vi "02_ui_plot_window.vi"() -> ()   [LabVIEW 2025]
uses:
  4c7a61b9-d50a-4fa5-8b88-644507a3af04.vi
  74ea501e-f43b-483f-8511-84a735437533.vi
  166e0385-1291-4ee6-a608-8b02bdaae3d2.vi
  b1158e5f-e22e-42fa-9d41-9ea4e4d0b9e3.vi
  31b119fa-27fe-4ebe-809c-2da1a8fd4d96.vi
  13143f16-a64c-4a8d-9511-2945b8db9dc5.vi
  9c1d92a2-1c85-4809-97a6-d36bf52cbad7.vi
  d684625a-03c4-4daf-8e9e-674a236ebb3e.vi
  fb960f78-e1fe-4b5d-8417-6d8be925c5cf.vi
  c135c75a-78bf-4448-8d92-d4bbbd51cd11.vi
  <vilib>/Utility/config.llb/Read Key (U32).vi
  <vilib>/Utility/config.llb/Read Key (Boolean).vi
  <vilib>/Utility/config.llb/Read Key (String).vi
  <vilib>/Utility/config.llb/Write Key (U32).vi
  <vilib>/Utility/config.llb/Write Key (Boolean).vi
  <vilib>/Utility/config.llb/Write Key (String).vi
  00_global_variables.vi
  <vilib>/Utility/config.llb/NI_LVConfig.lvlib
panel:
  out "loaded_config_path":path
  out "loaded_config_filename":string caption="Recent File"
  in  "open_config_plot_0":bool
  in  "safe_config_as_plot_0":bool
  in  "safe_config_plot_0":bool
  in  "select_plot_5":string(combo)="2"
  in  "select_plot_4":string(combo)="2"
  out "cursor_p5_1_prefix":string
  out "cursor_p4_1_prefix":string
  out "cursor_p5_2_prefix":string
  out "cursor_p4_2_prefix":string
  out "cursor_p5_2":dbl format="%#_6f"
  in  "color_picker_5":u32(colorbox)=14811391
  out "cursor_p5_1":dbl format="%#_6f"
  in  "enable_plot_5":bool caption="S11 - Imaginary"
  out "cursor_p4_2":dbl format="%#_6f"
  in  "color_picker_4":u32(colorbox)=49352
  out "cursor_p4_1":dbl format="%#_6f"
  in  "enable_plot_4":bool caption="S11 - Imaginary"
  in  "select_plot_3":string(combo)="2"
  in  "select_plot_2":string(combo)="2"
  in  "select_plot_1":string(combo)="2"
  in  "select_plot_0":string(combo)="2"
  out "cursor_p3_1_prefix":string
  out "cursor_p2_1_prefix":string
  out "cursor_p1_1_prefix":string
  out "cursor_p0_1_prefix":string
  out "cursor_p3_2_prefix":string
  out "cursor_p2_2_prefix":string
  out "cursor_p1_2_prefix":string
  out "cursor_p0_2_prefix":string
  out "cursor_p3_2":dbl format="%#_6f"
  in  "color_picker_3":u32(colorbox)=14468608
  out "cursor_p3_1":dbl format="%#_6f"
  in  "enable_plot_3":bool caption="S11 - Imaginary"
  out "cursor_p2_2":dbl format="%#_6f"
  in  "color_picker_2":u32(colorbox)=39219
  out "cursor_p2_1":dbl format="%#_6f"
  in  "enable_plot_2":bool caption="S11 - Imaginary"
  out "cursor_p1_2":dbl format="%#_6f"
  out "cursor_p0_2":dbl format="%#_6f"
  out "cursor_p0_freq_2":string caption="Frequenz"
  out "cursor_p0_wavel_2":dbl caption="Frequenz"
  out "cursor_p0_wavel_1":dbl caption="Frequenz"
  in  "color_picker_1":u32(colorbox)=14423100
  in  "color_picker_0":u32(colorbox)=26316
  out "cursor_p0_freq_1":string caption="Frequenz"
  out "cursor_p1_1":dbl format="%#_6f"
  out "cursor_p0_1":dbl format="%#_6f"
  in  "enable_plot_1":bool caption="S11 - Imaginary"
  in  "enable_plot_0":bool=TRUE
  out "plot_0":cluster{"array type (2D Dbl)":dbl[], dbl[]}[](graph)
  # "Cursor 2"
  # "Cursor 1"
  # "Hz"
  # "Frequency"
  # "Hz"
  # "Wavelength"
  # "m"
  # "m"
  # "Configuration"
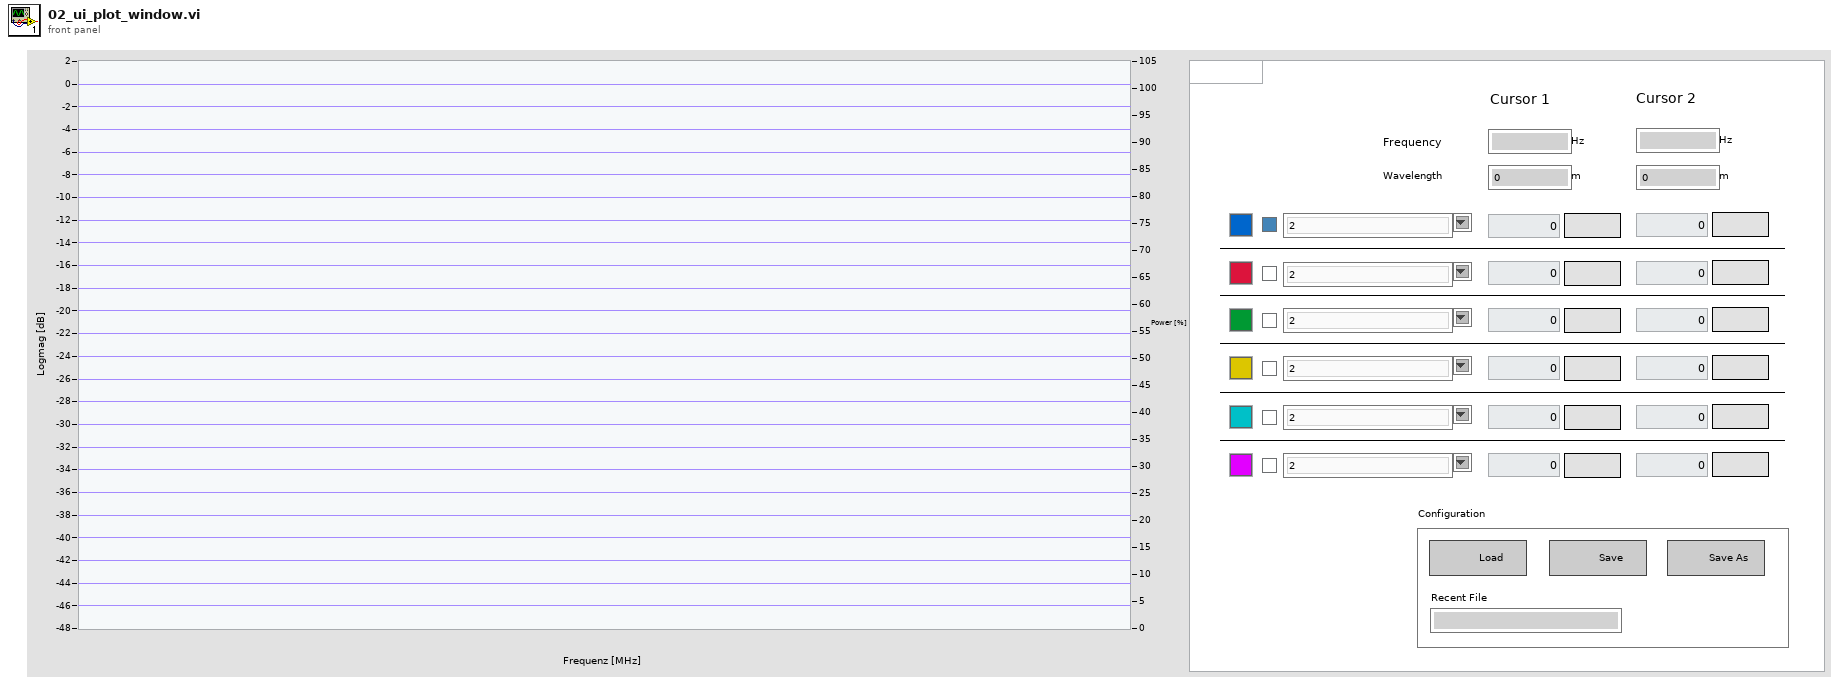
[diagram p1: front panel]
types:
  T1 = typedef "NI_LVConfig.lvlib/Config Data RefNum.ctl" = refnum<k1>
  T2 = typedef "LVComboBoxStrsAndValuesArrayTypeDef.ctl" = cluster{"String":string, "Value":string}[]
  T3 = cluster{"freq_array":dbl[], "data_array":dbl[]}[]
  T4 = cluster{"y_scale_id":u32, "unit":string, "prefix_enable":bool, "plot_id":u32}[]
  T5 = cluster{"y_scale_id":u32, "unit":string, "prefix_enable":bool, "plot_id":u32}
  T6 = typedef "LVCursorListTypeDef.ctl" = cluster{"Name":string, "Color":u32, "Style":u8, "Point Style":u8, "Name Visible":bool, "Allow Drag":bool, "Cursor Mode":u32, "Plot":i32, "Index":i32, "Position":cluster{"X":dbl, "Y":dbl}, "X Scale":u32, "Y Scale":u32, "Watch Plots":i32[], "Watch All Plots":bool, "Plot Area":i32, "Label Offset":cluster{"X":dbl, "Y":dbl}}[]
  T7 = cluster{"cursor_data":dbl[], "frequency":string, "wavelength_m":dbl}
  T8 = cluster{"cursor_0_color":u32, "cursor_1_color":u32}
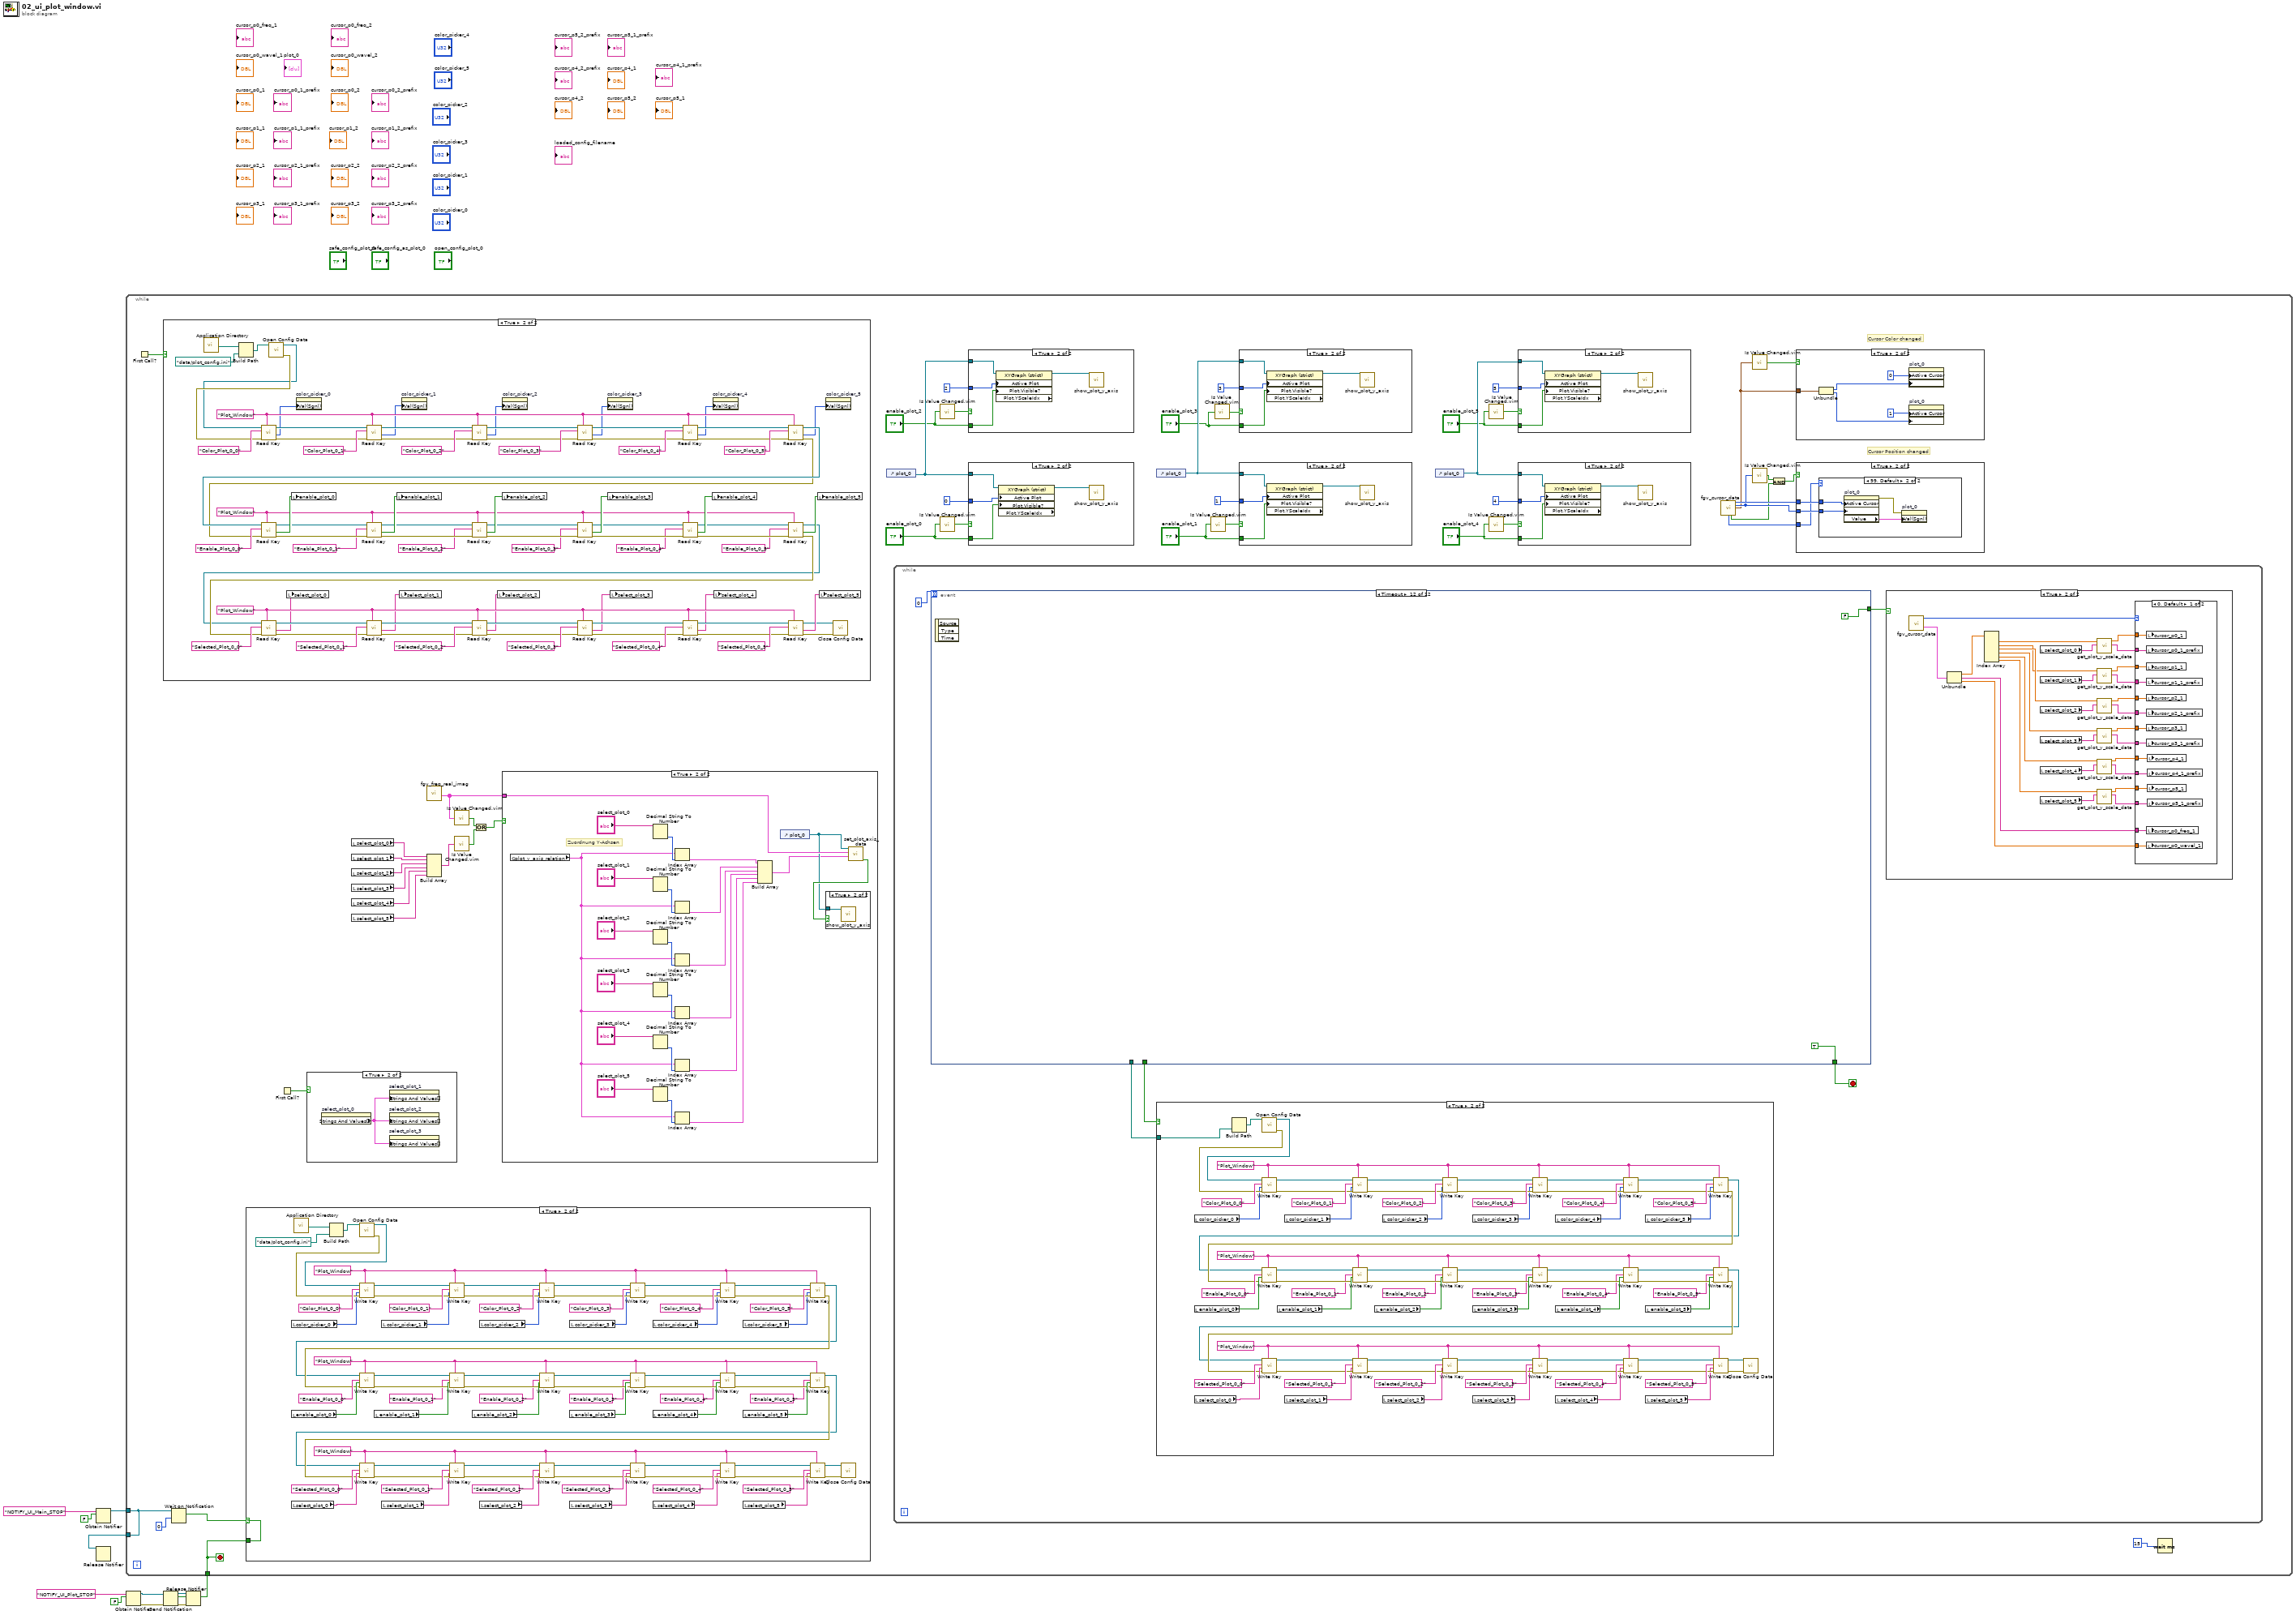
[diagram p0: block diagram]
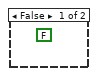
[diagram p11: hidden frame]
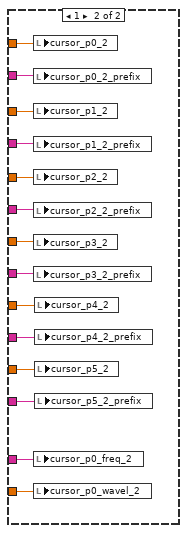
[diagram p18: hidden frame]
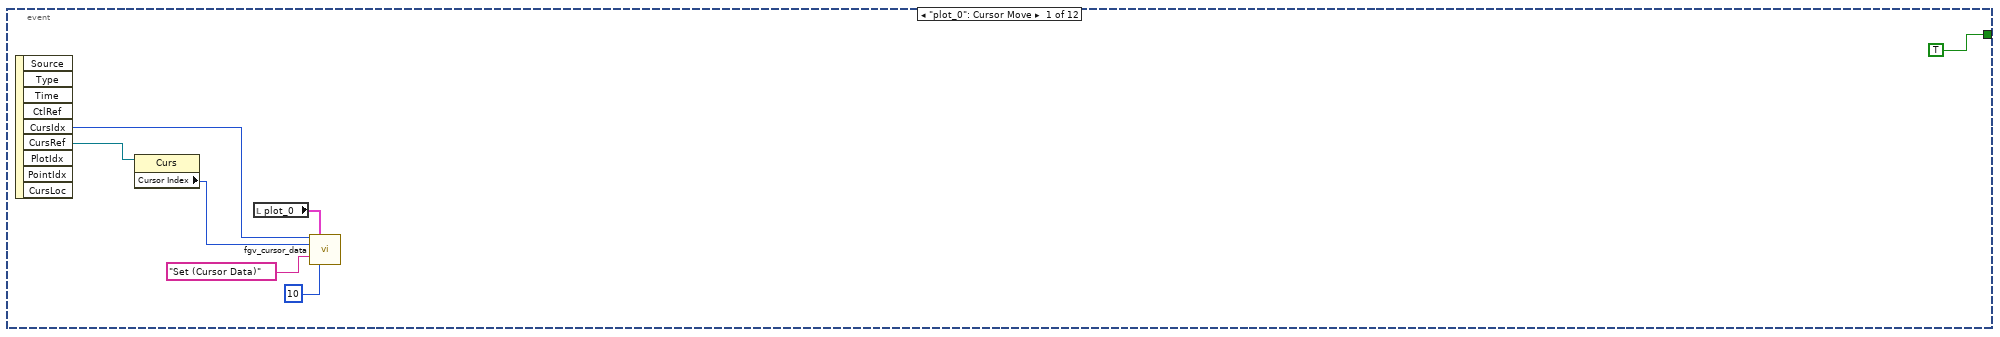
[diagram p19: hidden frame]
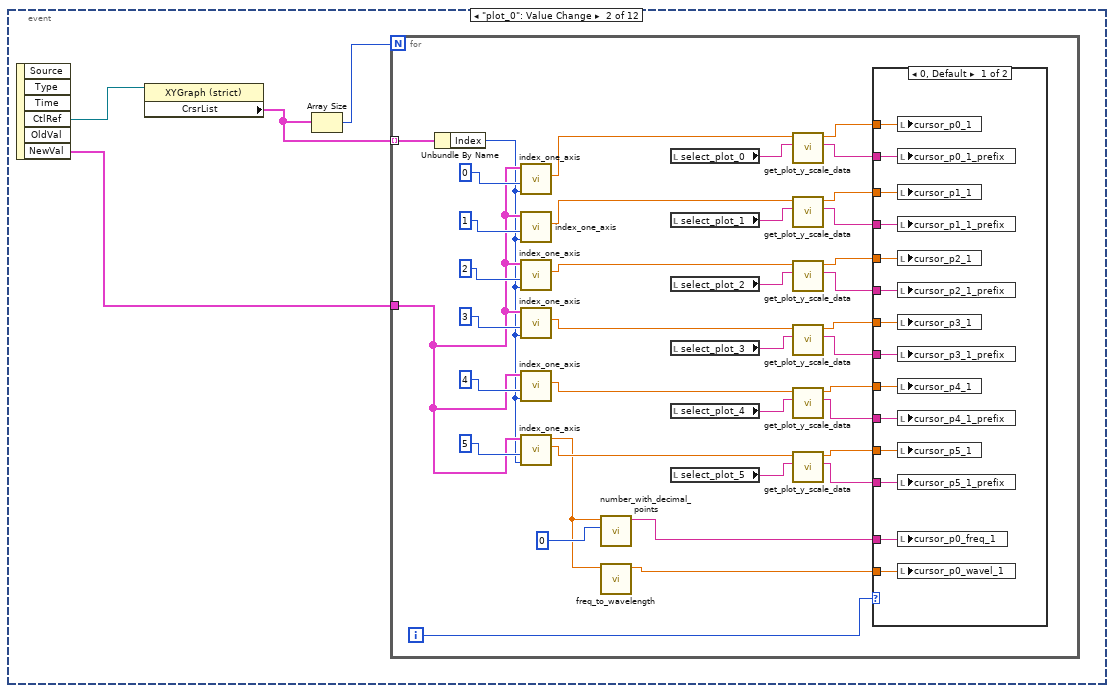
[diagram p20: hidden frame]
diagram:
  n1 = Obtain Notifier(name (unnamed)="NOTIFY_UI_Main_STOP", notification data type=FALSE) -> (notifier out=w9:refnum<notifier>)  [unwired: 2 in, 2 out]
  n2 = while {
    tunnel: w9 -> [w35]
    tunnel: [w35] -> w8
    tunnel: [w21] -> w1
    stop <- w21 stop-if-true
    # "Cursor Color changed"
    # "Cursor Position changed"
    n3 = First Call?() -> (First Call?: T/F=w20:bool)
    n4 = case shown="True" w20 {
      frame False {
      }
      frame True {
        w173 = "Plot_Window" ("section")
        w208 = "Plot_Window" ("section")
        w215 = "Plot_Window" ("section")
        n5 = call <vilib>:"Application Directory.vi"() -> ("Application Directory"=w158:path)
        n6 = Build Path(base path=w158, name or relative path=path "data/plot_config.ini") -> (appended path=w164:path)
        n7 = call <vilib>:"Open Config Data.vi"("configuration file path"=w164) -> ("error out"=w162:errorcluster, "refnum"=w161:T1)  [unwired: 8 in, 1 out]
        n8 = call-poly <vilib>:"Read Key.vi"("section"=w215, "error in (no error)"=w162, "key"="Color_Plot_0_0", "refnum"=w161) -> ("error out"=w228:errorcluster, "value"=w157:u32, "refnum out"=w229:T1)  [unwired: 4 in, 1 out]
        n9 = property on="color_picker_0" class="ColBox"("Val(Sgnl)"=w157) -> ()  [unwired: 2 in, 2 out]
        n10 = call-poly <vilib>:"Read Key.vi"("section"=w215, "error in (no error)"=w228, "key"="Color_Plot_0_1", "refnum"=w229) -> ("error out"=w225:errorcluster, "value"=w156:u32, "refnum out"=w226:T1)  [unwired: 4 in, 1 out]
        n11 = property on="color_picker_1" class="ColBox"("Val(Sgnl)"=w156) -> ()  [unwired: 2 in, 2 out]
        n12 = call-poly <vilib>:"Read Key.vi"("section"=w215, "error in (no error)"=w225, "key"="Color_Plot_0_2", "refnum"=w226) -> ("error out"=w222:errorcluster, "value"=w152:u32, "refnum out"=w223:T1)  [unwired: 4 in, 1 out]
        n13 = property on="color_picker_2" class="ColBox"("Val(Sgnl)"=w152) -> ()  [unwired: 2 in, 2 out]
        n14 = call-poly <vilib>:"Read Key.vi"("section"=w215, "error in (no error)"=w222, "key"="Color_Plot_0_3", "refnum"=w223) -> ("error out"=w219:errorcluster, "value"=w153:u32, "refnum out"=w220:T1)  [unwired: 4 in, 1 out]
        n15 = property on="color_picker_3" class="ColBox"("Val(Sgnl)"=w153) -> ()  [unwired: 2 in, 2 out]
        n16 = call-poly <vilib>:"Read Key.vi"("section"=w215, "error in (no error)"=w219, "key"="Color_Plot_0_4", "refnum"=w220) -> ("error out"=w217:errorcluster, "value"=w154:u32, "refnum out"=w216:T1)  [unwired: 4 in, 1 out]
        n17 = property on="color_picker_4" class="ColBox"("Val(Sgnl)"=w154) -> ()  [unwired: 2 in, 2 out]
        n18 = call-poly <vilib>:"Read Key.vi"("section"=w215, "error in (no error)"=w217, "key"="Color_Plot_0_5", "refnum"=w216) -> ("error out"=w190:errorcluster, "value"=w155:u32, "refnum out"=w191:T1)  [unwired: 4 in, 1 out]
        n19 = call-poly <vilib>:"Read Key.vi"("section"=w208, "error in (no error)"=w190, "key"="Enable_Plot_0_0", "refnum"=w191) -> ("error out"=w195:errorcluster, "value"=w209:bool, "refnum out"=w194:T1)  [unwired: 4 in, 1 out]
        n20 = local write "enable_plot_0"(w209) -> ()
        n21 = call-poly <vilib>:"Read Key.vi"("section"=w208, "error in (no error)"=w195, "key"="Enable_Plot_0_1", "refnum"=w194) -> ("error out"=w198:errorcluster, "value"=w210:bool, "refnum out"=w197:T1)  [unwired: 4 in, 1 out]
        n22 = local write "enable_plot_1"(w210) -> ()
        n23 = call-poly <vilib>:"Read Key.vi"("section"=w208, "error in (no error)"=w198, "key"="Enable_Plot_0_2", "refnum"=w197) -> ("error out"=w201:errorcluster, "value"=w211:bool, "refnum out"=w200:T1)  [unwired: 4 in, 1 out]
        n24 = local write "enable_plot_2"(w211) -> ()
        n25 = call-poly <vilib>:"Read Key.vi"("section"=w208, "error in (no error)"=w201, "key"="Enable_Plot_0_3", "refnum"=w200) -> ("error out"=w204:errorcluster, "value"=w212:bool, "refnum out"=w203:T1)  [unwired: 4 in, 1 out]
        n26 = local write "enable_plot_3"(w212) -> ()
        n27 = call-poly <vilib>:"Read Key.vi"("section"=w208, "error in (no error)"=w204, "key"="Enable_Plot_0_4", "refnum"=w203) -> ("error out"=w206:errorcluster, "value"=w213:bool, "refnum out"=w207:T1)  [unwired: 4 in, 1 out]
        n28 = local write "enable_plot_4"(w213) -> ()
        n29 = call-poly <vilib>:"Read Key.vi"("section"=w208, "error in (no error)"=w206, "key"="Enable_Plot_0_5", "refnum"=w207) -> ("error out"=w166:errorcluster, "value"=w214:bool, "refnum out"=w165:T1)  [unwired: 4 in, 1 out]
        n30 = call-poly <vilib>:"Read Key.vi"("section"=w173, "error in (no error)"=w166, "key"="Selected_Plot_0_0", "refnum"=w165) -> ("error out"=w186:errorcluster, "value"=w172:string, "refnum out"=w187:T1)  [unwired: 4 in, 1 out]
        n31 = local write "select_plot_0"(w172) -> ()
        n32 = call-poly <vilib>:"Read Key.vi"("section"=w173, "error in (no error)"=w186, "key"="Selected_Plot_0_1", "refnum"=w187) -> ("error out"=w183:errorcluster, "value"=w171:string, "refnum out"=w184:T1)  [unwired: 4 in, 1 out]
        n33 = local write "select_plot_1"(w171) -> ()
        n34 = call-poly <vilib>:"Read Key.vi"("section"=w173, "error in (no error)"=w183, "key"="Selected_Plot_0_2", "refnum"=w184) -> ("error out"=w180:errorcluster, "value"=w170:string, "refnum out"=w181:T1)  [unwired: 4 in, 1 out]
        n35 = local write "select_plot_2"(w170) -> ()
        n36 = call-poly <vilib>:"Read Key.vi"("section"=w173, "error in (no error)"=w180, "key"="Selected_Plot_0_3", "refnum"=w181) -> ("error out"=w177:errorcluster, "value"=w169:string, "refnum out"=w178:T1)  [unwired: 4 in, 1 out]
        n37 = local write "select_plot_3"(w169) -> ()
        n38 = call-poly <vilib>:"Read Key.vi"("section"=w173, "error in (no error)"=w177, "key"="Selected_Plot_0_4", "refnum"=w178) -> ("error out"=w175:errorcluster, "value"=w168:string, "refnum out"=w174:T1)  [unwired: 4 in, 1 out]
        n39 = local write "select_plot_4"(w168) -> ()
        n40 = call-poly <vilib>:"Read Key.vi"("section"=w173, "error in (no error)"=w175, "key"="Selected_Plot_0_5", "refnum"=w174) -> ("error out"=w159:errorcluster, "value"=w167:string, "refnum out"=w160:T1)  [unwired: 4 in, 1 out]
        n41 = local write "enable_plot_5"(w214) -> ()
        n42 = local write "select_plot_5"(w167) -> ()
        n43 = property on="color_picker_5" class="ColBox"("Val(Sgnl)"=w155) -> ()  [unwired: 2 in, 2 out]
        n44 = call <vilib>:"Close Config Data.vi"("error in (no error)"=w159, "refnum"=w160) -> ()  [unwired: 8 in, 2 out]
      }
    }
    n45 = Wait on Notification(notifier=w35, timeout in ms (-1)=0) -> (notification=w22:bool)  [unwired: 2 in, 3 out]
    n46 = case shown="True" w22 {
      selector: w22 -> [_ w151]
      tunnel: [_ w151] -> w21
      frame False {
      }
      frame True {
        w78 = "Plot_Window" ("section")
        w123 = "Plot_Window" ("section")
        w72 = "Plot_Window" ("section")
        n47 = local read "color_picker_0"() -> (w130:u32)
        n48 = local read "enable_plot_0"() -> (w118:bool)
        n49 = local read "select_plot_0"() -> (w83:string)
        n50 = call <vilib>:"Application Directory.vi"() -> ("Application Directory"=w71:path)
        n51 = Build Path(base path=w71, name or relative path=path "data/plot_config.ini") -> (appended path=w137:path)
        n52 = call <vilib>:"Open Config Data.vi"("configuration file path"=w137) -> ("error out"=w135:errorcluster, "refnum"=w134:T1)  [unwired: 8 in, 1 out]
        n53 = call-poly <vilib>:"Write Key.vi"("section"=w72, "error in (no error)"=w135, "value"=w130, "key"="Color_Plot_0_0", "refnum"=w134) -> ("error out"=w147:errorcluster, "refnum out"=w148:T1)  [unwired: 4 in, 1 out]
        n54 = local read "enable_plot_1"() -> (w119:bool)
        n55 = local read "color_picker_1"() -> (w129:u32)
        n56 = local read "select_plot_1"() -> (w82:string)
        n57 = call-poly <vilib>:"Write Key.vi"("section"=w72, "error in (no error)"=w147, "value"=w129, "key"="Color_Plot_0_1", "refnum"=w148) -> ("error out"=w144:errorcluster, "refnum out"=w145:T1)  [unwired: 4 in, 1 out]
        n58 = local read "enable_plot_2"() -> (w120:bool)
        n59 = local read "color_picker_2"() -> (w128:u32)
        n60 = local read "select_plot_2"() -> (w81:string)
        n61 = call-poly <vilib>:"Write Key.vi"("section"=w72, "error in (no error)"=w144, "value"=w128, "key"="Color_Plot_0_2", "refnum"=w145) -> ("error out"=w141:errorcluster, "refnum out"=w142:T1)  [unwired: 4 in, 1 out]
        n62 = local read "color_picker_3"() -> (w125:u32)
        n63 = local read "enable_plot_3"() -> (w124:bool)
        n64 = local read "select_plot_3"() -> (w77:string)
        n65 = call-poly <vilib>:"Write Key.vi"("section"=w72, "error in (no error)"=w141, "value"=w125, "key"="Color_Plot_0_3", "refnum"=w142) -> ("error out"=w138:errorcluster, "refnum out"=w139:T1)  [unwired: 4 in, 1 out]
        n66 = local read "color_picker_4"() -> (w127:u32)
        n67 = local read "enable_plot_4"() -> (w121:bool)
        n68 = local read "select_plot_4"() -> (w80:string)
        n69 = call-poly <vilib>:"Write Key.vi"("section"=w72, "error in (no error)"=w138, "value"=w127, "key"="Color_Plot_0_4", "refnum"=w139) -> ("error out"=w131:errorcluster, "refnum out"=w132:T1)  [unwired: 4 in, 1 out]
        n70 = local read "color_picker_5"() -> (w126:u32)
        n71 = local read "enable_plot_5"() -> (w122:bool)
        n72 = local read "select_plot_5"() -> (w79:string)
        n73 = call-poly <vilib>:"Write Key.vi"("section"=w72, "error in (no error)"=w131, "value"=w126, "key"="Color_Plot_0_5", "refnum"=w132) -> ("error out"=w101:errorcluster, "refnum out"=w100:T1)  [unwired: 4 in, 1 out]
        n74 = call-poly <vilib>:"Write Key.vi"("section"=w123, "error in (no error)"=w101, "value"=w118, "key"="Enable_Plot_0_0", "refnum"=w100) -> ("error out"=w105:errorcluster, "refnum out"=w104:T1)  [unwired: 4 in, 1 out]
        n75 = call-poly <vilib>:"Write Key.vi"("section"=w123, "error in (no error)"=w105, "value"=w119, "key"="Enable_Plot_0_1", "refnum"=w104) -> ("error out"=w108:errorcluster, "refnum out"=w107:T1)  [unwired: 4 in, 1 out]
        n76 = call-poly <vilib>:"Write Key.vi"("section"=w123, "error in (no error)"=w108, "value"=w120, "key"="Enable_Plot_0_2", "refnum"=w107) -> ("error out"=w111:errorcluster, "refnum out"=w110:T1)  [unwired: 4 in, 1 out]
        n77 = call-poly <vilib>:"Write Key.vi"("section"=w123, "error in (no error)"=w111, "value"=w124, "key"="Enable_Plot_0_3", "refnum"=w110) -> ("error out"=w114:errorcluster, "refnum out"=w113:T1)  [unwired: 4 in, 1 out]
        n78 = call-poly <vilib>:"Write Key.vi"("section"=w123, "error in (no error)"=w114, "value"=w121, "key"="Enable_Plot_0_4", "refnum"=w113) -> ("error out"=w117:errorcluster, "refnum out"=w116:T1)  [unwired: 4 in, 1 out]
        n79 = call-poly <vilib>:"Write Key.vi"("section"=w123, "error in (no error)"=w117, "value"=w122, "key"="Enable_Plot_0_5", "refnum"=w116) -> ("error out"=w76:errorcluster, "refnum out"=w75:T1)  [unwired: 4 in, 1 out]
        n80 = call-poly <vilib>:"Write Key.vi"("section"=w78, "error in (no error)"=w76, "value"=w83, "key"="Selected_Plot_0_0", "refnum"=w75) -> ("error out"=w96:errorcluster, "refnum out"=w97:T1)  [unwired: 4 in, 1 out]
        n81 = call-poly <vilib>:"Write Key.vi"("section"=w78, "error in (no error)"=w96, "value"=w82, "key"="Selected_Plot_0_1", "refnum"=w97) -> ("error out"=w93:errorcluster, "refnum out"=w94:T1)  [unwired: 4 in, 1 out]
        n82 = call-poly <vilib>:"Write Key.vi"("section"=w78, "error in (no error)"=w93, "value"=w81, "key"="Selected_Plot_0_2", "refnum"=w94) -> ("error out"=w90:errorcluster, "refnum out"=w91:T1)  [unwired: 4 in, 1 out]
        n83 = call-poly <vilib>:"Write Key.vi"("section"=w78, "error in (no error)"=w90, "value"=w77, "key"="Selected_Plot_0_3", "refnum"=w91) -> ("error out"=w87:errorcluster, "refnum out"=w88:T1)  [unwired: 4 in, 1 out]
        n84 = call-poly <vilib>:"Write Key.vi"("section"=w78, "error in (no error)"=w87, "value"=w80, "key"="Selected_Plot_0_4", "refnum"=w88) -> ("error out"=w84:errorcluster, "refnum out"=w85:T1)  [unwired: 4 in, 1 out]
        n85 = call-poly <vilib>:"Write Key.vi"("section"=w78, "error in (no error)"=w84, "value"=w79, "key"="Selected_Plot_0_5", "refnum"=w85) -> ("error out"=w73:errorcluster, "refnum out"=w74:T1)  [unwired: 4 in, 1 out]
        n86 = call <vilib>:"Close Config Data.vi"("error in (no error)"=w73, "refnum"=w74) -> ()  [unwired: 8 in, 2 out]
      }
    }
    n87 = First Call?() -> (First Call?: T/F=w32:bool)
    n88 = case shown="True" w32 {
      frame False {
      }
      frame True {
        n89 = property on="select_plot_0" class="CmbBox"() -> ("Strings And Values[]"=w240:T2)  [unwired: 2 in, 2 out]
        n90 = property on="select_plot_1" class="CmbBox"("Strings And Values[]"=w240) -> ()  [unwired: 2 in, 2 out]
        n91 = property on="select_plot_2" class="CmbBox"("Strings And Values[]"=w240) -> ()  [unwired: 2 in, 2 out]
        n92 = property on="select_plot_3" class="CmbBox"("Strings And Values[]"=w240) -> ()  [unwired: 2 in, 2 out]
      }
    }
    n93 = local read "select_plot_0"() -> (w47:string)
    n94 = local read "select_plot_1"() -> (w46:string)
    n95 = local read "select_plot_2"() -> (w45:string)
    n96 = local read "select_plot_3"() -> (w44:string)
    n97 = local read "select_plot_4"() -> (w24:string)
    n98 = local read "select_plot_5"() -> (w23:string)
    n99 = call "fgv_freq_real_imag.vi"() -> ("plot_data"=w33:T3)  [unwired: 8 in, 3 out]
    n100 = Build Array(w47, w46, w45, w44, w24, w23) -> (w43:string[])
    n101 = call "Is Value Changed.vim"("value"=w33) -> ("changed or first call?"=w48:bool)
    n102 = call "Is Value Changed.vim"("value"=w43) -> ("changed or first call?"=w42:bool)
    n103 = Or(x=w48, y=w42) -> (x .or. y?=w49:bool)
    n104 = case shown="True" w49 {
      tunnel: w33 -> [_ w259]
      frame False {
        (unwired) FALSE
      }
      frame True {
        # "Zuordnung Y-Achsen"
        n105 = global read "00_global_variables.vi" "plot_y_axis_relation"() -> (w247:T4)
        n106 = Decimal String To Number(string="select_plot_0") -> (number=w263:i32)  [unwired: 2 in, 1 out]
        n107 = Decimal String To Number(string="select_plot_1") -> (number=w262:i32)  [unwired: 2 in, 1 out]
        n108 = Decimal String To Number(string="select_plot_2") -> (number=w261:i32)  [unwired: 2 in, 1 out]
        n109 = Decimal String To Number(string="select_plot_3") -> (number=w260:i32)  [unwired: 2 in, 1 out]
        n110 = Decimal String To Number(string="select_plot_4") -> (number=w251:i32)  [unwired: 2 in, 1 out]
        n111 = Decimal String To Number(string="select_plot_5") -> (number=w250:i32)  [unwired: 2 in, 1 out]
        n112 = Index Array(array=w247, index=w263) -> (element=w256:T5)
        n113 = Index Array(array=w247, index=w262) -> (element=w255:T5)
        n114 = Index Array(array=w247, index=w261) -> (element=w254:T5)
        n115 = Index Array(array=w247, index=w260) -> (element=w253:T5)
        n116 = Index Array(array=w247, index=w251) -> (element=w246:T5)
        n117 = Index Array(array=w247, index=w250) -> (element=w245:T5)
        n118 = Build Array(w256, w255, w254, w253, w246, w245) -> (w252:T4)
        n119 = control-ref of="plot_0"() -> (w257:refnum<vi>)
        n120 = call "set_plot_axis_data.vi"("plot_allocation"=w252, "plot_data"=w259, "reference"=w257) -> ("done"=w258:bool)  [unwired: 8 in]
        n121 = case shown="True" w258 {
          tunnel: w257 -> [_ w268]
          frame False {
          }
          frame True {
            n122 = call "show_plot_y_axis.vi"("plot_ref_in"=w268) -> ()  [unwired: 9 in, 2 out]
          }
        }
      }
    }
    n123 = control-ref of="plot_0"() -> (w51:refnum<vi>)
    n124 = while {
      stop <- w285 stop-if-true
      n125 = event shown="[11] Timeout" {
        selector: _ -> [_ _ _ _ _ _ _ _ _ _ _ _]
        dyn-events: _ -> [_ _ _ _ _ _ _ _ _ _ _ _]
        timeout: 0 -> [_ _ _ _ _ _ _ _ _ _ _ _]
        tunnel: [_ _ _ _ _ _ _ _ _ _ _ TRUE] -> w285
        tunnel: [TRUE _ _ _ _ _ _ _ _ _ _ FALSE] -> w283
        tunnel: [_ _ _ _ _ _ _ _ _ w601 w623 _] -> w282
        tunnel: [_ _ _ _ _ _ _ _ _ w600 w622 _] -> w281
        event "plot_0": Cursor Move {
          n126 = event-data() -> ("CursIdx"=w428:i32, "CursRef"=w424:refnum<vi>)  [unwired: 1 in, 7 out]
          n127 = property on="Property Node" class="Curs"(reference=w424) -> ("Cursor Index"=w423:i32)  [unwired: 1 in, 2 out]
          n128 = local read "plot_0"() -> (w426:cluster{"array type (2D Dbl)":dbl[], dbl[]}[])
          n129 = call "fgv_cursor_data.vi"("cursor_idx_set"=w428, "plot_data_set"=w426, "cursor_pos_set"=w423, "mode"="Set (Cursor Data)", "plot_id_set"=10) -> ()  [unwired: 4 in, 7 out]
        }
        event "plot_0": Value Change {
          n130 = event-data() -> ("CtlRef"=w430:refnum<vi>, "NewVal"=w429:cluster{"array type (2D Dbl)":dbl[], dbl[]}[])  [unwired: 1 in, 4 out]
          n131 = property on="Property Node" class="XYGraph (strict)"(reference=w430) -> ("CrsrList"=w432:T6)  [unwired: 1 in, 2 out]
          n132 = Array Size(array=w432) -> (size(s)=w431:i32)
          n133 = for {
            N: w431 -> [_]
            tunnel: w432 -> [w470] mode=indexing
            tunnel: w429 -> [w439]
            i -> [w452]
            n134 = Unbundle By Name(w470) -> ("Index"=w438:i32)
            n135 = call "index_one_axis.vi"("x_index"=w438, "curve_sel"=0 ("x_index"), "graph_data"=w439) -> ("Y"=w449:dbl)  [unwired: 7 in, 1 out]
            n136 = call "index_one_axis.vi"("x_index"=w438, "curve_sel"=1 ("x_index"), "graph_data"=w439) -> ("Y"=w448:dbl)  [unwired: 7 in, 1 out]
            n137 = call "index_one_axis.vi"("x_index"=w438, "curve_sel"=2 ("x_index"), "graph_data"=w439) -> ("Y"=w447:dbl)  [unwired: 7 in, 1 out]
            n138 = call "index_one_axis.vi"("x_index"=w438, "curve_sel"=3 ("x_index"), "graph_data"=w439) -> ("Y"=w446:dbl)  [unwired: 7 in, 1 out]
            n139 = call "index_one_axis.vi"("x_index"=w438, "curve_sel"=4 ("x_index"), "graph_data"=w439) -> ("Y"=w445:dbl)  [unwired: 7 in, 1 out]
            n140 = call "index_one_axis.vi"("x_index"=w438, "curve_sel"=5 ("x_index"), "graph_data"=w439) -> ("Y"=w440:dbl, "X"=w437:dbl)  [unwired: 7 in]
            n141 = call "number_with_decimal_points.vi"("Precision"=i16 0, "Double"=w437) -> ("String"=w450:string)  [unwired: 5 in]
            n142 = call "freq_to_wavelength.vi"("frequency_hz"=w437) -> ("wavelength_m"=w451:dbl)  [unwired: 10 in]
            n143 = local read "select_plot_0"() -> (w464:string)
            n144 = local read "select_plot_1"() -> (w463:string)
            n145 = local read "select_plot_2"() -> (w462:string)
            n146 = local read "select_plot_3"() -> (w455:string)
            n147 = local read "select_plot_4"() -> (w444:string)
            n148 = local read "select_plot_5"() -> (w441:string)
            n149 = call "get_plot_y_scale_data.vi"("plot_selector"=w464, "cursor_value_in"=w449) -> ("prefix/unit"=w459:string, "cursor_value_out"=w458:dbl)  [unwired: 8 in]
            n150 = call "get_plot_y_scale_data.vi"("plot_selector"=w463, "cursor_value_in"=w448) -> ("prefix/unit"=w460:string, "cursor_value_out"=w457:dbl)  [unwired: 8 in]
            n151 = call "get_plot_y_scale_data.vi"("plot_selector"=w462, "cursor_value_in"=w447) -> ("prefix/unit"=w461:string, "cursor_value_out"=w456:dbl)  [unwired: 8 in]
            n152 = call "get_plot_y_scale_data.vi"("plot_selector"=w455, "cursor_value_in"=w446) -> ("prefix/unit"=w453:string, "cursor_value_out"=w454:dbl)  [unwired: 8 in]
            n153 = call "get_plot_y_scale_data.vi"("plot_selector"=w444, "cursor_value_in"=w445) -> ("prefix/unit"=w434:string, "cursor_value_out"=w433:dbl)  [unwired: 8 in]
            n154 = call "get_plot_y_scale_data.vi"("plot_selector"=w441, "cursor_value_in"=w440) -> ("prefix/unit"=w436:string, "cursor_value_out"=w435:dbl)  [unwired: 8 in]
            n155 = case shown="0, Default" w452 {
              tunnel: w458 -> [w484 w498]
              tunnel: w457 -> [w483 w497]
              tunnel: w456 -> [w482 w496]
              tunnel: w454 -> [w481 w495]
              tunnel: w450 -> [w480 w494]
              tunnel: w451 -> [w479 w493]
              tunnel: w453 -> [w478 w489]
              tunnel: w459 -> [w477 w492]
              tunnel: w460 -> [w476 w491]
              tunnel: w461 -> [w475 w490]
              tunnel: w436 -> [w474 w485]
              tunnel: w435 -> [w473 w486]
              tunnel: w434 -> [w472 w487]
              tunnel: w433 -> [w471 w488]
              frame 0, Default {
                n156 = local write "cursor_p0_1"(w484) -> ()
                n157 = local write "cursor_p0_1_prefix"(w477) -> ()
                n158 = local write "cursor_p1_1"(w483) -> ()
                n159 = local write "cursor_p1_1_prefix"(w476) -> ()
                n160 = local write "cursor_p2_1"(w482) -> ()
                n161 = local write "cursor_p2_1_prefix"(w475) -> ()
                n162 = local write "cursor_p3_1"(w481) -> ()
                n163 = local write "cursor_p3_1_prefix"(w478) -> ()
                n164 = local write "cursor_p4_1"(w471) -> ()
                n165 = local write "cursor_p4_1_prefix"(w472) -> ()
                n166 = local write "cursor_p5_1"(w473) -> ()
                n167 = local write "cursor_p5_1_prefix"(w474) -> ()
                n168 = local write "cursor_p0_freq_1"(w480) -> ()
                n169 = local write "cursor_p0_wavel_1"(w479) -> ()
              }
              frame 1 {
                n170 = local write "cursor_p0_2"(w498) -> ()
                n171 = local write "cursor_p0_2_prefix"(w492) -> ()
                n172 = local write "cursor_p1_2"(w497) -> ()
                n173 = local write "cursor_p1_2_prefix"(w491) -> ()
                n174 = local write "cursor_p2_2"(w496) -> ()
                n175 = local write "cursor_p2_2_prefix"(w490) -> ()
                n176 = local write "cursor_p3_2"(w495) -> ()
                n177 = local write "cursor_p3_2_prefix"(w489) -> ()
                n178 = local write "cursor_p4_2"(w488) -> ()
                n179 = local write "cursor_p4_2_prefix"(w487) -> ()
                n180 = local write "cursor_p5_2"(w486) -> ()
                n181 = local write "cursor_p5_2_prefix"(w485) -> ()
                n182 = local write "cursor_p0_freq_2"(w494) -> ()
                n183 = local write "cursor_p0_wavel_2"(w493) -> ()
              }
            }
          }
        }
        event "color_picker_0": Value Change {
          n184 = event-data() -> ("NewVal"=w499:u32)  [unwired: 1 in, 5 out]
          n185 = property on="plot_0" class="XYGraph (strict)"("Active Plot"=u32 0, "Plot.Plot Color"=w499) -> ()  [unwired: 2 in, 2 out]
        }
        event "color_picker_1": Value Change {
          n186 = event-data() -> ("NewVal"=w501:u32)  [unwired: 1 in, 5 out]
          n187 = property on="plot_0" class="XYGraph (strict)"("Active Plot"=u32 1, "Plot.Plot Color"=w501) -> ()  [unwired: 2 in, 2 out]
        }
        event "color_picker_2": Value Change {
          n188 = event-data() -> ("NewVal"=w503:u32)  [unwired: 1 in, 5 out]
          n189 = property on="plot_0" class="XYGraph (strict)"("Active Plot"=u32 2, "Plot.Plot Color"=w503) -> ()  [unwired: 2 in, 2 out]
        }
        event "color_picker_3": Value Change {
          n190 = event-data() -> ("NewVal"=w505:u32)  [unwired: 1 in, 5 out]
          n191 = property on="plot_0" class="XYGraph (strict)"("Active Plot"=u32 3, "Plot.Plot Color"=w505) -> ()  [unwired: 2 in, 2 out]
        }
        event "color_picker_4": Value Change {
          n192 = event-data() -> ("NewVal"=w507:u32)  [unwired: 1 in, 5 out]
          n193 = property on="plot_0" class="XYGraph (strict)"("Active Plot"=u32 4, "Plot.Plot Color"=w507) -> ()  [unwired: 2 in, 2 out]
        }
        event "color_picker_5": Value Change {
          n194 = event-data() -> ("NewVal"=w509:u32)  [unwired: 1 in, 5 out]
          n195 = property on="plot_0" class="XYGraph (strict)"("Active Plot"=u32 5, "Plot.Plot Color"=w509) -> ()  [unwired: 2 in, 2 out]
        }
        event "open_config_plot_0": Value Change {
          n196 = event-data() -> ("NewVal"=w511:bool)  [unwired: 1 in, 5 out]
          n197 = case shown="True" w511 {
            selector: w511 -> [_ w514]
            frame False {
            }
            frame True {
              n198 = Not(x=w514) -> (.not. x?=w513:bool)
              n199 = call "File Dialog2"("pattern (all files)"="*.ini" ("pattern label"), "pattern label"="INI-File") -> ("selected path"=w515:path, "cancelled"=w519:bool, "error out"=w512:errorcluster)  [unwired: 10 in, 1 out]
              n200 = local write "open_config_plot_0"(w513) -> ()
              n201 = Not(x=w519) -> (.not. x?=w516:bool)
              n202 = call <vilib>:"Clear Errors.vi"("error in (no error)"=w512) -> ()  [unwired: 5 in, 2 out]
              n203 = case shown="True" w516 {
                tunnel: w515 -> [_ w520]
                frame False {
                }
                frame True {
                  w541 = "Plot_Window" ("section")
                  w576 = "Plot_Window" ("section")
                  w583 = "Plot_Window" ("section")
                  n204 = Build Path(name or relative path=w520) -> (appended path=w532:path)  [unwired: 1 in]
                  n205 = call <vilib>:"Open Config Data.vi"("configuration file path"=w532) -> ("error out"=w531:errorcluster, "refnum"=w530:T1)  [unwired: 8 in, 1 out]
                  n206 = call-poly <vilib>:"Read Key.vi"("section"=w583, "error in (no error)"=w531, "key"="Color_Plot_0_0", "refnum"=w530) -> ("error out"=w596:errorcluster, "value"=w527:u32, "refnum out"=w597:T1)  [unwired: 4 in, 1 out]
                  n207 = property on="color_picker_0" class="ColBox"("Val(Sgnl)"=w527) -> ()  [unwired: 2 in, 2 out]
                  n208 = Strip Path(path=w520) -> (name=w521:string)  [unwired: 1 out]
                  n209 = local write "loaded_config_filename"(w521) -> ()
                  n210 = call-poly <vilib>:"Read Key.vi"("section"=w583, "error in (no error)"=w596, "key"="Color_Plot_0_1", "refnum"=w597) -> ("error out"=w593:errorcluster, "value"=w526:u32, "refnum out"=w594:T1)  [unwired: 4 in, 1 out]
                  n211 = property on="color_picker_1" class="ColBox"("Val(Sgnl)"=w526) -> ()  [unwired: 2 in, 2 out]
                  n212 = call-poly <vilib>:"Read Key.vi"("section"=w583, "error in (no error)"=w593, "key"="Color_Plot_0_2", "refnum"=w594) -> ("error out"=w590:errorcluster, "value"=w525:u32, "refnum out"=w591:T1)  [unwired: 4 in, 1 out]
                  n213 = property on="color_picker_2" class="ColBox"("Val(Sgnl)"=w525) -> ()  [unwired: 2 in, 2 out]
                  n214 = call-poly <vilib>:"Read Key.vi"("section"=w583, "error in (no error)"=w590, "key"="Color_Plot_0_3", "refnum"=w591) -> ("error out"=w587:errorcluster, "value"=w524:u32, "refnum out"=w588:T1)  [unwired: 4 in, 1 out]
                  n215 = property on="color_picker_3" class="ColBox"("Val(Sgnl)"=w524) -> ()  [unwired: 2 in, 2 out]
                  n216 = call-poly <vilib>:"Read Key.vi"("section"=w583, "error in (no error)"=w587, "key"="Color_Plot_0_4", "refnum"=w588) -> ("error out"=w585:errorcluster, "value"=w523:u32, "refnum out"=w584:T1)  [unwired: 4 in, 1 out]
                  n217 = property on="color_picker_4" class="ColBox"("Val(Sgnl)"=w523) -> ()  [unwired: 2 in, 2 out]
                  n218 = call-poly <vilib>:"Read Key.vi"("section"=w583, "error in (no error)"=w585, "key"="Color_Plot_0_5", "refnum"=w584) -> ("error out"=w558:errorcluster, "value"=w522:u32, "refnum out"=w559:T1)  [unwired: 4 in, 1 out]
                  n219 = call-poly <vilib>:"Read Key.vi"("section"=w576, "error in (no error)"=w558, "key"="Enable_Plot_0_0", "refnum"=w559) -> ("error out"=w563:errorcluster, "value"=w577:bool, "refnum out"=w562:T1)  [unwired: 4 in, 1 out]
                  n220 = local write "enable_plot_0"(w577) -> ()
                  n221 = call-poly <vilib>:"Read Key.vi"("section"=w576, "error in (no error)"=w563, "key"="Enable_Plot_0_1", "refnum"=w562) -> ("error out"=w566:errorcluster, "value"=w578:bool, "refnum out"=w565:T1)  [unwired: 4 in, 1 out]
                  n222 = local write "enable_plot_1"(w578) -> ()
                  n223 = call-poly <vilib>:"Read Key.vi"("section"=w576, "error in (no error)"=w566, "key"="Enable_Plot_0_2", "refnum"=w565) -> ("error out"=w569:errorcluster, "value"=w579:bool, "refnum out"=w568:T1)  [unwired: 4 in, 1 out]
                  n224 = local write "enable_plot_2"(w579) -> ()
                  n225 = call-poly <vilib>:"Read Key.vi"("section"=w576, "error in (no error)"=w569, "key"="Enable_Plot_0_3", "refnum"=w568) -> ("error out"=w572:errorcluster, "value"=w580:bool, "refnum out"=w571:T1)  [unwired: 4 in, 1 out]
                  n226 = local write "enable_plot_3"(w580) -> ()
                  n227 = call-poly <vilib>:"Read Key.vi"("section"=w576, "error in (no error)"=w572, "key"="Enable_Plot_0_4", "refnum"=w571) -> ("error out"=w574:errorcluster, "value"=w581:bool, "refnum out"=w575:T1)  [unwired: 4 in, 1 out]
                  n228 = local write "enable_plot_4"(w581) -> ()
                  n229 = call-poly <vilib>:"Read Key.vi"("section"=w576, "error in (no error)"=w574, "key"="Enable_Plot_0_5", "refnum"=w575) -> ("error out"=w534:errorcluster, "value"=w582:bool, "refnum out"=w533:T1)  [unwired: 4 in, 1 out]
                  n230 = call-poly <vilib>:"Read Key.vi"("section"=w541, "error in (no error)"=w534, "key"="Selected_Plot_0_0", "refnum"=w533) -> ("error out"=w554:errorcluster, "value"=w540:string, "refnum out"=w555:T1)  [unwired: 4 in, 1 out]
                  n231 = local write "select_plot_0"(w540) -> ()
                  n232 = call-poly <vilib>:"Read Key.vi"("section"=w541, "error in (no error)"=w554, "key"="Selected_Plot_0_1", "refnum"=w555) -> ("error out"=w551:errorcluster, "value"=w539:string, "refnum out"=w552:T1)  [unwired: 4 in, 1 out]
                  n233 = local write "select_plot_1"(w539) -> ()
                  n234 = call-poly <vilib>:"Read Key.vi"("section"=w541, "error in (no error)"=w551, "key"="Selected_Plot_0_2", "refnum"=w552) -> ("error out"=w548:errorcluster, "value"=w538:string, "refnum out"=w549:T1)  [unwired: 4 in, 1 out]
                  n235 = local write "select_plot_2"(w538) -> ()
                  n236 = call-poly <vilib>:"Read Key.vi"("section"=w541, "error in (no error)"=w548, "key"="Selected_Plot_0_3", "refnum"=w549) -> ("error out"=w545:errorcluster, "value"=w537:string, "refnum out"=w546:T1)  [unwired: 4 in, 1 out]
                  n237 = local write "select_plot_3"(w537) -> ()
                  n238 = call-poly <vilib>:"Read Key.vi"("section"=w541, "error in (no error)"=w545, "key"="Selected_Plot_0_4", "refnum"=w546) -> ("error out"=w543:errorcluster, "value"=w536:string, "refnum out"=w542:T1)  [unwired: 4 in, 1 out]
                  n239 = local write "select_plot_4"(w536) -> ()
                  n240 = call-poly <vilib>:"Read Key.vi"("section"=w541, "error in (no error)"=w543, "key"="Selected_Plot_0_5", "refnum"=w542) -> ("error out"=w528:errorcluster, "value"=w535:string, "refnum out"=w529:T1)  [unwired: 4 in, 1 out]
                  n241 = local write "enable_plot_5"(w582) -> ()
                  n242 = property on="color_picker_5" class="ColBox"("Val(Sgnl)"=w522) -> ()  [unwired: 2 in, 2 out]
                  n243 = local write "select_plot_5"(w535) -> ()
                  n244 = call <vilib>:"Close Config Data.vi"("error in (no error)"=w528, "refnum"=w529) -> ()  [unwired: 8 in, 2 out]
                  "loaded_config_path" <- w520
                }
              }
            }
          }
        }
        event "safe_config_plot_0": Value Change {
          n245 = event-data() -> ("NewVal"=w602:bool)  [unwired: 1 in, 5 out]
          n246 = case shown="True" w602 {
            selector: w602 -> [_ w608]
            tunnel: [_ w604] -> w601
            tunnel: [_ w603] -> w600
            frame False {
            }
            frame True {
              n247 = local read "loaded_config_filename"() -> (w605:string)
              n248 = Not(x=w608) -> (.not. x?=w609:bool)
              n249 = local write "safe_config_plot_0"(w609) -> ()
              n250 = Not Equal?(x=w605, y="") -> (x != y?=w606:bool)
              n251 = case shown="False" w606 {
                tunnel: w605 -> [_ w621]
                tunnel: [w611 w618] -> w604
                tunnel: [w612 w617] -> w603
                frame False {
                  n252 = call "File Dialog3"("pattern (all files)"="*.ini" ("pattern label"), "pattern label"="INI-File") -> ("selected path"=w612:path, "cancelled"=w613:bool, "error out"=w610:errorcluster)  [unwired: 10 in, 1 out]
                  n253 = Not(x=w613) -> (.not. x?=w611:bool)
                  n254 = call <vilib>:"Clear Errors.vi"("error in (no error)"=w610) -> ()  [unwired: 5 in, 2 out]
                }
                frame True {
                  n255 = local read "loaded_config_path"() -> (w617:path)
                  n256 = Concatenate Strings(w621, " will be overwritten!" ("string")) -> (w619:string)
                  n257 = call "Display Message to User"("Message"=w619) -> ("error out"=w616:errorcluster, "OK"=w618:bool)  [unwired: 9 in]
                  n258 = call <vilib>:"Clear Errors.vi"("error in (no error)"=w616) -> ()  [unwired: 5 in, 2 out]
                }
              }
            }
          }
        }
        event "safe_config_as_plot_0": Value Change {
          n259 = event-data() -> ("NewVal"=w624:bool)  [unwired: 1 in, 5 out]
          n260 = case shown="True" w624 {
            selector: w624 -> [_ w628]
            tunnel: [_ w627] -> w623
            tunnel: [_ w626] -> w622
            frame False {
            }
            frame True {
              n261 = Not(x=w628) -> (.not. x?=w629:bool)
              n262 = local write "safe_config_as_plot_0"(w629) -> ()
              n263 = call "File Dialog"("pattern (all files)"="*.ini" ("pattern label"), "pattern label"="INI-File") -> ("selected path"=w626:path, "cancelled"=w630:bool, "error out"=w625:errorcluster)  [unwired: 10 in, 1 out]
              n264 = Not(x=w630) -> (.not. x?=w627:bool)
              n265 = call <vilib>:"Clear Errors.vi"("error in (no error)"=w625) -> ()  [unwired: 5 in, 2 out]
            }
          }
        }
        event Timeout {
          n266 = event-data() -> ()  [unwired: 1 in, 3 out]
        }
      }
      n267 = case shown="True" w282 {
        tunnel: w281 -> [_ w286]
        frame False {
        }
        frame True {
          w293 = "Plot_Window" ("section")
          w338 = "Plot_Window" ("section")
          w287 = "Plot_Window" ("section")
          n268 = local read "color_picker_0"() -> (w345:u32)
          n269 = local read "enable_plot_0"() -> (w333:bool)
          n270 = local read "select_plot_0"() -> (w298:string)
          n271 = Build Path(name or relative path=w286) -> (appended path=w351:path)  [unwired: 1 in]
          n272 = call <vilib>:"Open Config Data.vi"("configuration file path"=w351) -> ("error out"=w350:errorcluster, "refnum"=w349:T1)  [unwired: 8 in, 1 out]
          n273 = call-poly <vilib>:"Write Key.vi"("section"=w287, "error in (no error)"=w350, "value"=w345, "key"="Color_Plot_0_0", "refnum"=w349) -> ("error out"=w361:errorcluster, "refnum out"=w362:T1)  [unwired: 4 in, 1 out]
          n274 = local read "enable_plot_1"() -> (w334:bool)
          n275 = local read "color_picker_1"() -> (w344:u32)
          n276 = local read "select_plot_1"() -> (w297:string)
          n277 = call-poly <vilib>:"Write Key.vi"("section"=w287, "error in (no error)"=w361, "value"=w344, "key"="Color_Plot_0_1", "refnum"=w362) -> ("error out"=w358:errorcluster, "refnum out"=w359:T1)  [unwired: 4 in, 1 out]
          n278 = local read "enable_plot_2"() -> (w335:bool)
          n279 = local read "color_picker_2"() -> (w343:u32)
          n280 = local read "select_plot_2"() -> (w296:string)
          n281 = call-poly <vilib>:"Write Key.vi"("section"=w287, "error in (no error)"=w358, "value"=w343, "key"="Color_Plot_0_2", "refnum"=w359) -> ("error out"=w355:errorcluster, "refnum out"=w356:T1)  [unwired: 4 in, 1 out]
          n282 = local read "color_picker_3"() -> (w340:u32)
          n283 = local read "enable_plot_3"() -> (w339:bool)
          n284 = local read "select_plot_3"() -> (w292:string)
          n285 = call-poly <vilib>:"Write Key.vi"("section"=w287, "error in (no error)"=w355, "value"=w340, "key"="Color_Plot_0_3", "refnum"=w356) -> ("error out"=w352:errorcluster, "refnum out"=w353:T1)  [unwired: 4 in, 1 out]
          n286 = local read "color_picker_4"() -> (w342:u32)
          n287 = local read "enable_plot_4"() -> (w336:bool)
          n288 = local read "select_plot_4"() -> (w295:string)
          n289 = call-poly <vilib>:"Write Key.vi"("section"=w287, "error in (no error)"=w352, "value"=w342, "key"="Color_Plot_0_4", "refnum"=w353) -> ("error out"=w346:errorcluster, "refnum out"=w347:T1)  [unwired: 4 in, 1 out]
          n290 = local read "color_picker_5"() -> (w341:u32)
          n291 = local read "enable_plot_5"() -> (w337:bool)
          n292 = local read "select_plot_5"() -> (w294:string)
          n293 = call-poly <vilib>:"Write Key.vi"("section"=w287, "error in (no error)"=w346, "value"=w341, "key"="Color_Plot_0_5", "refnum"=w347) -> ("error out"=w316:errorcluster, "refnum out"=w315:T1)  [unwired: 4 in, 1 out]
          n294 = call-poly <vilib>:"Write Key.vi"("section"=w338, "error in (no error)"=w316, "value"=w333, "key"="Enable_Plot_0_0", "refnum"=w315) -> ("error out"=w320:errorcluster, "refnum out"=w319:T1)  [unwired: 4 in, 1 out]
          n295 = call-poly <vilib>:"Write Key.vi"("section"=w338, "error in (no error)"=w320, "value"=w334, "key"="Enable_Plot_0_1", "refnum"=w319) -> ("error out"=w323:errorcluster, "refnum out"=w322:T1)  [unwired: 4 in, 1 out]
          n296 = call-poly <vilib>:"Write Key.vi"("section"=w338, "error in (no error)"=w323, "value"=w335, "key"="Enable_Plot_0_2", "refnum"=w322) -> ("error out"=w326:errorcluster, "refnum out"=w325:T1)  [unwired: 4 in, 1 out]
          n297 = call-poly <vilib>:"Write Key.vi"("section"=w338, "error in (no error)"=w326, "value"=w339, "key"="Enable_Plot_0_3", "refnum"=w325) -> ("error out"=w329:errorcluster, "refnum out"=w328:T1)  [unwired: 4 in, 1 out]
          n298 = call-poly <vilib>:"Write Key.vi"("section"=w338, "error in (no error)"=w329, "value"=w336, "key"="Enable_Plot_0_4", "refnum"=w328) -> ("error out"=w332:errorcluster, "refnum out"=w331:T1)  [unwired: 4 in, 1 out]
          n299 = call-poly <vilib>:"Write Key.vi"("section"=w338, "error in (no error)"=w332, "value"=w337, "key"="Enable_Plot_0_5", "refnum"=w331) -> ("error out"=w291:errorcluster, "refnum out"=w290:T1)  [unwired: 4 in, 1 out]
          n300 = call-poly <vilib>:"Write Key.vi"("section"=w293, "error in (no error)"=w291, "value"=w298, "key"="Selected_Plot_0_0", "refnum"=w290) -> ("error out"=w311:errorcluster, "refnum out"=w312:T1)  [unwired: 4 in, 1 out]
          n301 = call-poly <vilib>:"Write Key.vi"("section"=w293, "error in (no error)"=w311, "value"=w297, "key"="Selected_Plot_0_1", "refnum"=w312) -> ("error out"=w308:errorcluster, "refnum out"=w309:T1)  [unwired: 4 in, 1 out]
          n302 = call-poly <vilib>:"Write Key.vi"("section"=w293, "error in (no error)"=w308, "value"=w296, "key"="Selected_Plot_0_2", "refnum"=w309) -> ("error out"=w305:errorcluster, "refnum out"=w306:T1)  [unwired: 4 in, 1 out]
          n303 = call-poly <vilib>:"Write Key.vi"("section"=w293, "error in (no error)"=w305, "value"=w292, "key"="Selected_Plot_0_3", "refnum"=w306) -> ("error out"=w302:errorcluster, "refnum out"=w303:T1)  [unwired: 4 in, 1 out]
          n304 = call-poly <vilib>:"Write Key.vi"("section"=w293, "error in (no error)"=w302, "value"=w295, "key"="Selected_Plot_0_4", "refnum"=w303) -> ("error out"=w299:errorcluster, "refnum out"=w300:T1)  [unwired: 4 in, 1 out]
          n305 = call-poly <vilib>:"Write Key.vi"("section"=w293, "error in (no error)"=w299, "value"=w294, "key"="Selected_Plot_0_5", "refnum"=w300) -> ("error out"=w288:errorcluster, "refnum out"=w289:T1)  [unwired: 4 in, 1 out]
          n306 = call <vilib>:"Close Config Data.vi"("error in (no error)"=w288, "refnum"=w289) -> ()  [unwired: 8 in, 2 out]
        }
      }
      n307 = case shown="True" w283 {
        frame False {
        }
        frame True {
          n308 = call "fgv_cursor_data.vi"() -> ("cursor_idx_get"=w393:i32, "cursor_data_get"=w365:T7)  [unwired: 9 in, 5 out]
          n309 = Unbundle(w365) -> ("cursor_data"=w392:dbl[], "frequency"=w391:string, "wavelength_m"=w390:dbl)
          n310 = Index Array(array=w392) -> (element #1=w381:dbl, element #2=w383:dbl, element #3=w385:dbl, element #4=w386:dbl, element #5=w371:dbl, element #6=w370:dbl)  [unwired: 6 in]
          n311 = local read "select_plot_0"() -> (w374:string)
          n312 = local read "select_plot_1"() -> (w375:string)
          n313 = local read "select_plot_2"() -> (w376:string)
          n314 = local read "select_plot_3"() -> (w387:string)
          n315 = local read "select_plot_4"() -> (w373:string)
          n316 = local read "select_plot_5"() -> (w372:string)
          n317 = call "get_plot_y_scale_data.vi"("plot_selector"=w374, "cursor_value_in"=w381) -> ("prefix/unit"=w379:string, "cursor_value_out"=w380:dbl)  [unwired: 8 in]
          n318 = call "get_plot_y_scale_data.vi"("plot_selector"=w375, "cursor_value_in"=w383) -> ("prefix/unit"=w378:string, "cursor_value_out"=w382:dbl)  [unwired: 8 in]
          n319 = call "get_plot_y_scale_data.vi"("plot_selector"=w376, "cursor_value_in"=w385) -> ("prefix/unit"=w377:string, "cursor_value_out"=w384:dbl)  [unwired: 8 in]
          n320 = call "get_plot_y_scale_data.vi"("plot_selector"=w387, "cursor_value_in"=w386) -> ("prefix/unit"=w389:string, "cursor_value_out"=w388:dbl)  [unwired: 8 in]
          n321 = call "get_plot_y_scale_data.vi"("plot_selector"=w373, "cursor_value_in"=w371) -> ("prefix/unit"=w369:string, "cursor_value_out"=w368:dbl)  [unwired: 8 in]
          n322 = call "get_plot_y_scale_data.vi"("plot_selector"=w372, "cursor_value_in"=w370) -> ("prefix/unit"=w367:string, "cursor_value_out"=w366:dbl)  [unwired: 8 in]
          n323 = case shown="0, Default" w393 {
            tunnel: w380 -> [w407 w421]
            tunnel: w382 -> [w406 w419]
            tunnel: w384 -> [w405 w417]
            tunnel: w388 -> [w404 w415]
            tunnel: w391 -> [w403 w413]
            tunnel: w390 -> [w402 w412]
            tunnel: w389 -> [w401 w414]
            tunnel: w379 -> [w400 w420]
            tunnel: w378 -> [w399 w418]
            tunnel: w377 -> [w398 w416]
            tunnel: w369 -> [w397 w410]
            tunnel: w368 -> [w396 w411]
            tunnel: w367 -> [w395 w408]
            tunnel: w366 -> [w394 w409]
            frame 0, Default {
              n324 = local write "cursor_p0_1"(w407) -> ()
              n325 = local write "cursor_p0_1_prefix"(w400) -> ()
              n326 = local write "cursor_p1_1"(w406) -> ()
              n327 = local write "cursor_p1_1_prefix"(w399) -> ()
              n328 = local write "cursor_p2_1"(w405) -> ()
              n329 = local write "cursor_p2_1_prefix"(w398) -> ()
              n330 = local write "cursor_p3_1"(w404) -> ()
              n331 = local write "cursor_p3_1_prefix"(w401) -> ()
              n332 = local write "cursor_p0_freq_1"(w403) -> ()
              n333 = local write "cursor_p0_wavel_1"(w402) -> ()
              n334 = local write "cursor_p4_1"(w396) -> ()
              n335 = local write "cursor_p4_1_prefix"(w397) -> ()
              n336 = local write "cursor_p5_1"(w394) -> ()
              n337 = local write "cursor_p5_1_prefix"(w395) -> ()
            }
            frame 1 {
              n338 = local write "cursor_p0_2"(w421) -> ()
              n339 = local write "cursor_p0_2_prefix"(w420) -> ()
              n340 = local write "cursor_p1_2"(w419) -> ()
              n341 = local write "cursor_p1_2_prefix"(w418) -> ()
              n342 = local write "cursor_p2_2"(w417) -> ()
              n343 = local write "cursor_p2_2_prefix"(w416) -> ()
              n344 = local write "cursor_p3_2"(w415) -> ()
              n345 = local write "cursor_p3_2_prefix"(w414) -> ()
              n346 = local write "cursor_p0_freq_2"(w413) -> ()
              n347 = local write "cursor_p0_wavel_2"(w412) -> ()
              n348 = local write "cursor_p4_2"(w411) -> ()
              n349 = local write "cursor_p4_2_prefix"(w410) -> ()
              n350 = local write "cursor_p5_2"(w409) -> ()
              n351 = local write "cursor_p5_2_prefix"(w408) -> ()
            }
          }
        }
      }
    }
    n352 = call "Is Value Changed.vim"("value"="enable_plot_2") -> ("changed or first call?"=w53:bool)
    n353 = call "Is Value Changed.vim"("value"="enable_plot_0") -> ("changed or first call?"=w36:bool)
    n354 = case shown="True" w53 {
      tunnel: "enable_plot_2" -> [_ w269]
      tunnel: w51 -> [_ w272]
      tunnel: 2 ("plot_id") -> [_ w271]
      frame False {
      }
      frame True {
        n355 = property on="Property Node" class="XYGraph (strict)" props=["Active Plot", "Plot", "Visible?", "Plot", "YScaleIdx"](reference=w272, "Active Plot"=w271, "Plot.Visible?"=w269) -> (reference out=w270:refnum<vi>)  [unwired: 1 in, 2 out]
        n356 = call "show_plot_y_axis.vi"("plot_ref_in"=w270) -> ()  [unwired: 9 in, 2 out]
      }
    }
    n357 = case shown="True" w36 {
      tunnel: "enable_plot_0" -> [_ w278]
      tunnel: w51 -> [_ w280]
      tunnel: 0 ("plot_id") -> [_ w279]
      frame False {
      }
      frame True {
        n358 = property on="Property Node" class="XYGraph (strict)" props=["Active Plot", "Plot", "Visible?", "Plot", "YScaleIdx"](reference=w280, "Active Plot"=w279, "Plot.Visible?"=w278) -> (reference out=w277:refnum<vi>)  [unwired: 1 in, 2 out]
        n359 = call "show_plot_y_axis.vi"("plot_ref_in"=w277) -> ()  [unwired: 9 in, 2 out]
      }
    }
    n360 = control-ref of="plot_0"() -> (w41:refnum<vi>)
    n361 = call "Is Value Changed.vim"("value"="enable_plot_1") -> ("changed or first call?"=w56:bool)
    n362 = call "Is Value Changed.vim"("value"="enable_plot_3") -> ("changed or first call?"=w39:bool)
    n363 = case shown="True" w39 {
      tunnel: "enable_plot_3" -> [_ w241]
      tunnel: w41 -> [_ w244]
      tunnel: 3 ("plot_id") -> [_ w243]
      frame False {
      }
      frame True {
        n364 = property on="Property Node" class="XYGraph (strict)" props=["Active Plot", "Plot", "Visible?", "Plot", "YScaleIdx"](reference=w244, "Active Plot"=w243, "Plot.Visible?"=w241) -> (reference out=w242:refnum<vi>)  [unwired: 1 in, 2 out]
        n365 = call "show_plot_y_axis.vi"("plot_ref_in"=w242) -> ()  [unwired: 9 in, 2 out]
      }
    }
    n366 = case shown="True" w56 {
      tunnel: "enable_plot_1" -> [_ w273]
      tunnel: w41 -> [_ w276]
      tunnel: 1 ("plot_id") -> [_ w275]
      frame False {
      }
      frame True {
        n367 = property on="Property Node" class="XYGraph (strict)" props=["Active Plot", "Plot", "Visible?", "Plot", "YScaleIdx"](reference=w276, "Active Plot"=w275, "Plot.Visible?"=w273) -> (reference out=w274:refnum<vi>)  [unwired: 1 in, 2 out]
        n368 = call "show_plot_y_axis.vi"("plot_ref_in"=w274) -> ()  [unwired: 9 in, 2 out]
      }
    }
    n369 = control-ref of="plot_0"() -> (w26:refnum<vi>)
    n370 = call "Is Value Changed.vim"("value"="enable_plot_5") -> ("changed or first call?"=w28:bool)
    n371 = call "Is Value Changed.vim"("value"="enable_plot_4") -> ("changed or first call?"=w31:bool)
    n372 = case shown="True" w28 {
      tunnel: "enable_plot_5" -> [_ w232]
      tunnel: w26 -> [_ w235]
      tunnel: 5 ("plot_id") -> [_ w234]
      frame False {
      }
      frame True {
        n373 = property on="Property Node" class="XYGraph (strict)" props=["Active Plot", "Plot", "Visible?", "Plot", "YScaleIdx"](reference=w235, "Active Plot"=w234, "Plot.Visible?"=w232) -> (reference out=w233:refnum<vi>)  [unwired: 1 in, 2 out]
        n374 = call "show_plot_y_axis.vi"("plot_ref_in"=w233) -> ()  [unwired: 9 in, 2 out]
      }
    }
    n375 = case shown="True" w31 {
      tunnel: "enable_plot_4" -> [_ w236]
      tunnel: w26 -> [_ w239]
      tunnel: 4 ("plot_id") -> [_ w238]
      frame False {
      }
      frame True {
        n376 = property on="Property Node" class="XYGraph (strict)" props=["Active Plot", "Plot", "Visible?", "Plot", "YScaleIdx"](reference=w239, "Active Plot"=w238, "Plot.Visible?"=w236) -> (reference out=w237:refnum<vi>)  [unwired: 1 in, 2 out]
        n377 = call "show_plot_y_axis.vi"("plot_ref_in"=w237) -> ()  [unwired: 9 in, 2 out]
      }
    }
    n378 = call "fgv_cursor_data.vi"() -> ("cursor_idx_get"=w19:i32, "cursor_pos_get"=w17:i32, "cursor_color_get"=w12:T8, "plot_id_get"=w18:i32, "cursor_mode_get"=w14:bool)  [unwired: 9 in, 2 out]
    n379 = call "Is Value Changed.vim"("value"=w12) -> ("changed or first call?"=w13:bool)
    n380 = call "Is Value Changed.vim"("value"=w17) -> ("changed or first call?"=w15:bool)
    n381 = And(x=w15, y=w14) -> (x .and. y?=w16:bool)
    n382 = case shown="True" w13 {
      tunnel: w12 -> [_ w63]
      frame False {
      }
      frame True {
        n383 = Unbundle(w63) -> ("cursor_0_color"=w59:u32, "cursor_1_color"=w60:u32)
        n384 = property on="plot_0" class="XYGraph (strict)"("Active Cursor"=u32 0, "Cursor.Cursor Color"=w59) -> ()  [unwired: 2 in, 2 out]
        n385 = property on="plot_0" class="XYGraph (strict)"("Active Cursor"=u32 1, "Cursor.Cursor Color"=w60) -> ()  [unwired: 2 in, 2 out]
      }
    }
    n386 = case shown="True" w16 {
      tunnel: w17 -> [_ w66]
      tunnel: w19 -> [_ w65]
      tunnel: w18 -> [_ w64]
      frame False {
      }
      frame True {
        n387 = case shown="99, Default" w64 {
          tunnel: w65 -> [_ w70]
          tunnel: w66 -> [_ w69]
          frame 10 {
          }
          frame 99, Default {
            n388 = property on="plot_0" class="XYGraph (strict)"("Active Cursor"=w70, "Cursor.Cursor Index"=w69) -> (error out=w67:errorcluster, "Value"=w68:cluster{"array type (2D Dbl)":dbl[], dbl[]}[])  [unwired: 2 in, 1 out]
            n389 = property on="plot_0" class="XYGraph (strict)"(error in=w67, "Val(Sgnl)"=w68) -> ()  [unwired: 1 in, 2 out]
          }
        }
      }
    }
    n390 = Wait (ms)(milliseconds to wait=u32 15) -> ()  [unwired: 1 out]
  }
  n391 = Release Notifier(notifier=w8) -> ()  [unwired: 2 in, 3 out]
  n392 = Obtain Notifier(name (unnamed)="NOTIFY_UI_Plot_STOP", notification data type=FALSE) -> (notifier out=w5:refnum<notifier>, error out=w4:errorcluster)  [unwired: 2 in, 1 out]
  n393 = Send Notification(notification=w1, notifier=w5, error in (no error)=w4) -> (notifier out=w3:refnum<notifier>, error out=w2:errorcluster)
  n394 = Release Notifier(notifier=w3, error in (no error)=w2) -> ()  [unwired: 1 in, 3 out]
